vi "DisconnectCore.vi"(8 "error in (no error)":errorcluster, 11 "GRPCClient in":refnum<class "MicronTemplateAPIs.lvclass">) -> (0 "error out":errorcluster, 3 "GRPCClient out":refnum<class "MicronTemplateAPIs.lvclass">)   [LabVIEW 2019, in "MicronTemplateAPIs.lvlib" / "MicronTemplateAPIs.lvclass"]
uses:
  MicronTemplateAPIs.lvclass
  gRPC/Client/MicronGRPCClient.lvclass
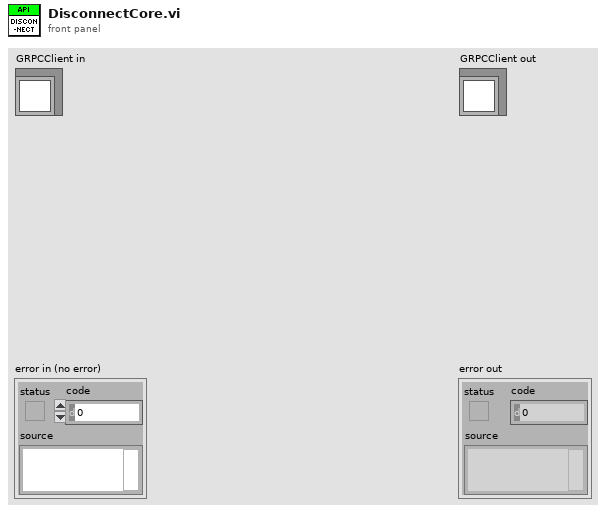
[diagram p1: front panel]
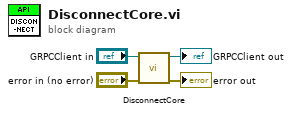
[diagram p0: block diagram]
diagram:
  n1 = call-parent "DisconnectCore.vi"("error in (no error)"="error in (no error)", "GRPCClient in"="GRPCClient in") -> ("error out"=→"error out":errorcluster, "GRPCClient out"=→"GRPCClient out":refnum<class "MicronTemplateAPIs.lvclass">)  [unwired: 8 in]
